vi "Get_MachineCode.vi"(8 "error in (no error)":errorcluster, 11 "Ref In":T1={"MS SQL Connection"=refnum, "UDL File"=path "", "Time"="", "DCODE"="", "WIP+1"=0, "MC No?"=0, "POKAYOKE?"=FALSE, "Expected Result"="", "Result [Status]"="", "Clock"=0.0, "RFID"="", "WIP Queue"=refnum, "TS Parameter"={"ProfitCenterCode"="", "LineCode"="", "WorkOrderNumber"="", "Model"="", "Model_with_Prefix"="", "VendorCode"="", "SetParameterDateCode"="", "PokaYoke"=0, "Target"=1, "Live_DateCode"="", "CustomerPartNumber"="", "Hand"="", "sBarcode"=FALSE, "FCA"=0, "Ent_Stamp"=timestamp(0 s since 1904-01-01), "STS_CD"=0.0}, "Data_Queue"=[], "RFID Serial No."=""} {"TS Parameter"."FCA" format="%01d"; "TS Parameter"."Target" min=1 max=100000; "TS Parameter"."PokaYoke" min=0 max=1}) -> (0 "error out":errorcluster, 1 "OperationCode":string[](array[string]), 2 "Machine Codes":string[](array[string]), 3 "Ref Out":T1={"MS SQL Connection"=refnum, "UDL File"=path "", "Time"="", "DCODE"="", "WIP+1"=0, "MC No?"=0, "POKAYOKE?"=FALSE, "Expected Result"="", "Result [Status]"="", "Clock"=0.0, "RFID"="", "WIP Queue"=refnum, "TS Parameter"={"ProfitCenterCode"="", "LineCode"="", "WorkOrderNumber"="", "Model"="", "Model_with_Prefix"="", "VendorCode"="", "SetParameterDateCode"="", "PokaYoke"=0, "Target"=1, "Live_DateCode"="", "CustomerPartNumber"="", "Hand"="", "sBarcode"=FALSE, "FCA"=0, "Ent_Stamp"=timestamp(0 s since 1904-01-01), "STS_CD"=0.0}, "Data_Queue"=[], "RFID Serial No."=""} {"TS Parameter"."FCA" format="%01d"; "TS Parameter"."Target" min=1 max=100000; "TS Parameter"."PokaYoke" min=0 max=1})   [LabVIEW 2020]
uses:
  Controls/TD SQL.ctl
  <vilib>/addons/database/Connection.llb/Conn ObjectReference.ctl
  Controls/WIP_State.ctl
  Controls/TS_Parameter.ctl
  <vilib>/regexp/Match Regular Expression.xnode
  <vilib>/addons/database/NI_Database_API.lvlib
panel:
  out "tables":string[](array[string])
  out "Array 2":string[](array[string])
  out "tables 2":string[](array[string])
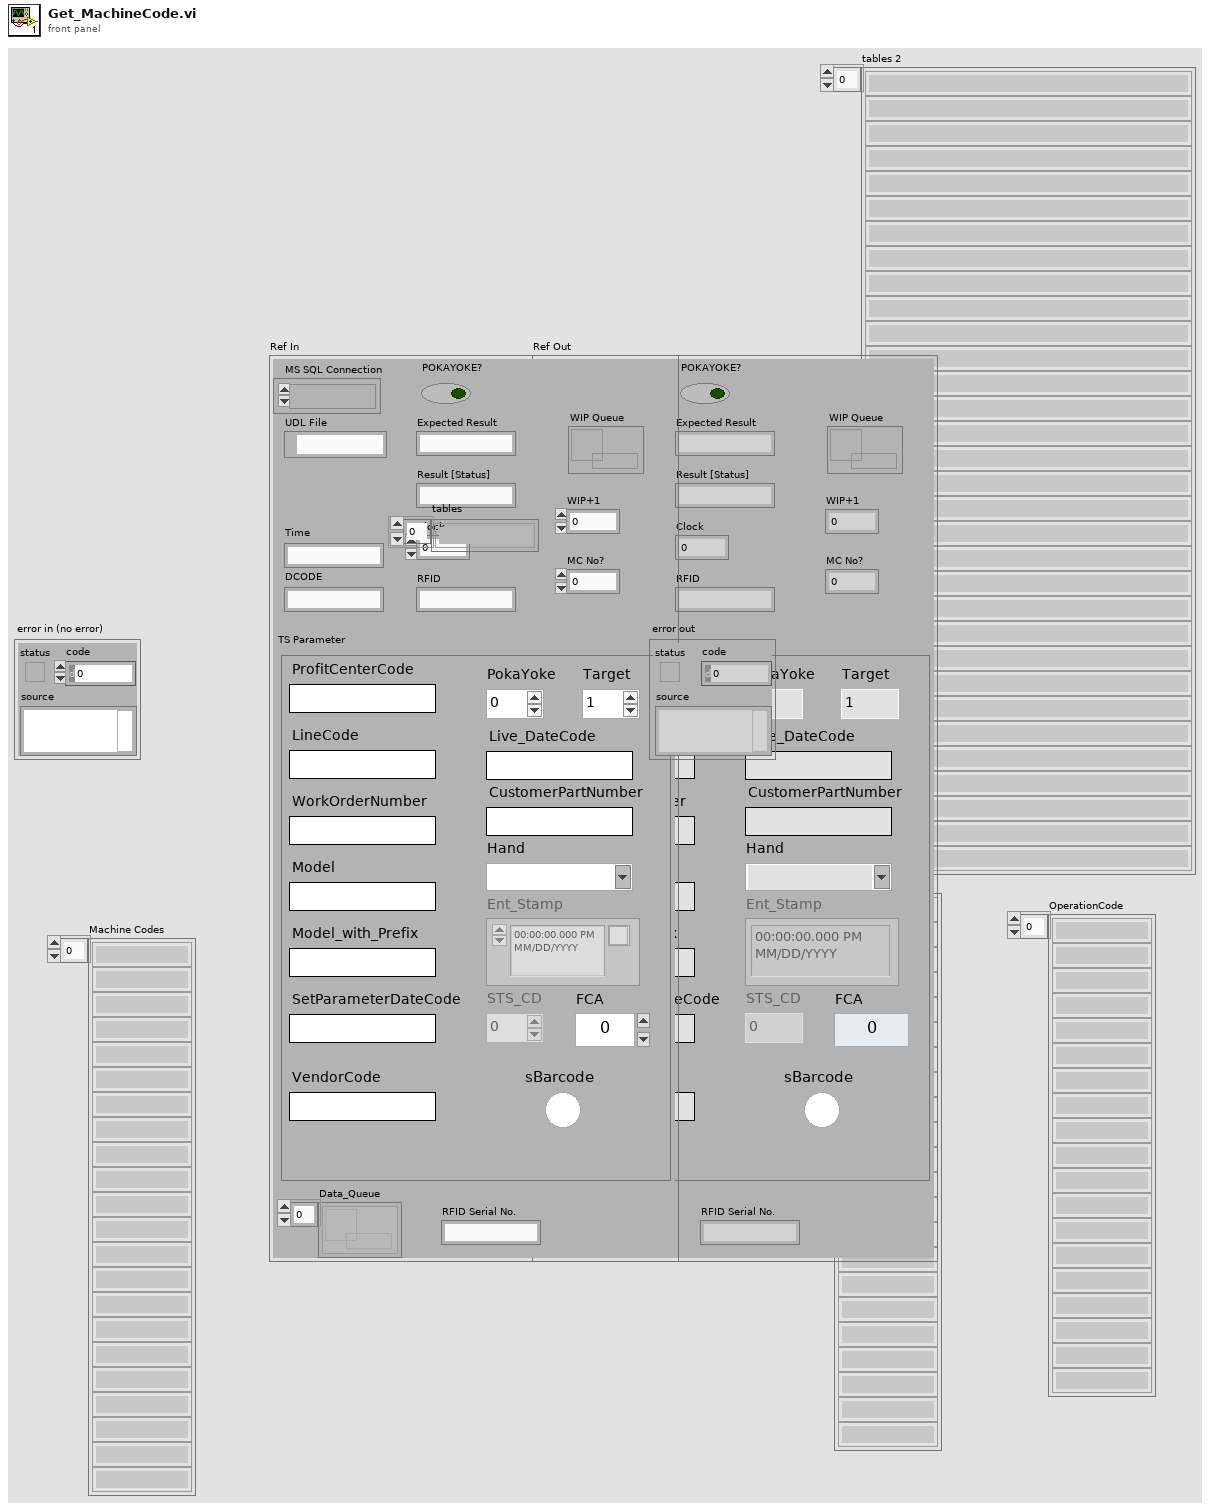
[diagram p1: front panel]
types:
  T1 = typedef "TD SQL.ctl" = cluster{"MS SQL Connection":T2, "UDL File":path, "Time":string, "DCODE":string, "WIP+1":i64, "MC No?":i32, "POKAYOKE?":bool, "Expected Result":string, "Result [Status]":string, "Clock":dbl, "RFID":string, "WIP Queue":refnum<queue>, "TS Parameter":T3, "Data_Queue":refnum<queue>[], "RFID Serial No.":string}
  T2 = typedef "NI_Database_API.lvlib/Conn ObjectReference.ctl" = refnum<k1>
  T3 = typedef "TS_Parameter.ctl" = cluster{"ProfitCenterCode":string, "LineCode":string, "WorkOrderNumber":string, "Model":string, "Model_with_Prefix":string, "VendorCode":string, "SetParameterDateCode":string, "PokaYoke":i32, "Target":i32, "Live_DateCode":string, "CustomerPartNumber":string, "Hand":string, "sBarcode":bool, "FCA":i32, "Ent_Stamp":timestamp, "STS_CD":dbl}
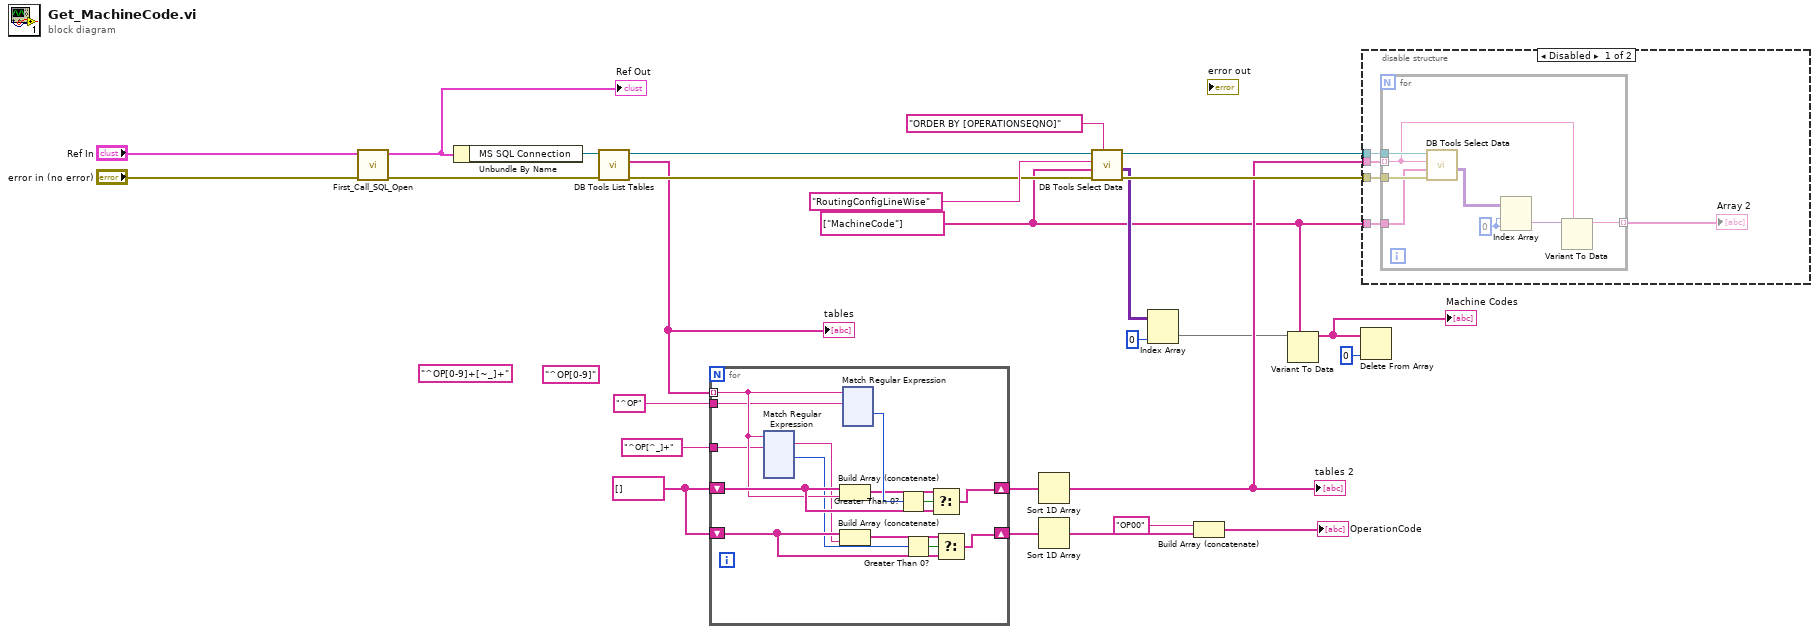
[diagram p0: block diagram]
diagram:
  (unwired) "^OP[0-9]" ("regular expression")
  (unwired) "^OP[0-9]+[~_]+" ("regular expression")
  w14 = string[] ["MachineCode"] ("columns")
  w6 = string[] [] ("tables")
  n1 = call "First_Call_SQL_Open.vi"("error in (no error)"="error in (no error)", "Ref In"="Ref In") -> ("error out"=w24:errorcluster, "Ref Out"=w26:T1)  [unwired: 8 in]
  "Ref Out" <- w26
  n2 = Unbundle By Name(w26) -> ("MS SQL Connection"=w25:T2)
  n3 = call <vilib>:"DB Tools List Tables.vi"("error in (no error)"=w24, "connection reference"=w25) -> ("error out"=w21:errorcluster, "tables"=w12:string[], "connection reference out"=w23:T2)  [unwired: 3 in]
  "tables" <- w12
  n4 = for {
    tunnel: w12 -> [w36] mode=indexing
    shift-right: [w37] -> w27
    shift-left: w6 -> [w38]
    tunnel: "^OP[^_]+" ("regular expression") -> [w35]
    shift-right: [w34] -> w5
    shift-left: w6 -> [w31]
    tunnel: "^OP" ("regular expression") -> [w28]
    n5 = xnode "Match Regular Expression"("input string"=w36, "regular expression"=w35) -> ("whole match"=w29:string, "offset past match"=w30:i32)  [unwired: 4 in, 4 out]
    n6 = Build Array (concatenate)(w38, w36) -> (w39:string[])
    n7 = Build Array (concatenate)(w31, w29) -> (w33:string[])
    n8 = xnode "Match Regular Expression"("input string"=w36, "regular expression"=w28) -> ("offset past match"=w41:i32)  [unwired: 4 in, 4 out]
    n9 = Greater Than 0?(x=w41) -> (x > 0?=w40:bool)
    n10 = Greater Than 0?(x=w30) -> (x > 0?=w32:bool)
    n11 = Select(t=w39, s=w40, f=w38) -> (s? t:f=w37:string[])
    n12 = Select(t=w33, s=w32, f=w31) -> (s? t:f=w34:string[])
  }
  n13 = Sort 1D Array(array=w27) -> (sorted array=w18:string[])
  "tables 2" <- w18
  n14 = Sort 1D Array(array=w5) -> (sorted array=w4:string[])
  n15 = call <vilib>:"DB Tools Select Data.vi"("condition"="ORDER BY [OPERATIONSEQNO]", "error in (no error)"=w21, "columns"=w14, "table"="RoutingConfigLineWise", "connection reference"=w23) -> ("error out"=w19:errorcluster, "data"=w16:variant[][], "connection reference out"=w20:T2)  [unwired: 1 in]
  n16 = Index Array(array=w16, index (col)=0 ("disabled index (col)")) -> (element=w15:variant[])  [unwired: 1 in]
  n17 = Build Array (concatenate)("OP00" ("String"), w4) -> (→"OperationCode":string[])
  n18 = Variant To Data(type=w14, Variant=w15) -> (data=w8:string[])  [unwired: 1 in, 1 out]
  "Machine Codes" <- w8
  n19 = Delete From Array(array=w8, index=0) -> ()  [unwired: 1 in, 2 out]
  n20 = disable-structure shown="Disabled" {
    disable-tunnel: w20 -> [w276 _]
    disable-tunnel: w19 -> [w275 _]
    disable-tunnel: w18 -> [w274 _]
    disable-tunnel: w14 -> [w273 _]
    frame Disabled {
      n21 = for {
        tunnel: w276 -> [w284]
        tunnel: w275 -> [w283]
        tunnel: w274 -> [w277] mode=indexing
        tunnel: w273 -> [w280]
        tunnel: [w279] -> w272 mode=indexing
        w278 = 0 ("disabled index (col)")
        n22 = call <vilib>:"DB Tools Select Data.vi"("error in (no error)"=w283, "columns"=w280, "table"=w277, "connection reference"=w284) -> ("data"=w282:variant[][])  [unwired: 2 in, 2 out]
        n23 = Index Array(array=w282, index (row)=w278, index (col)=w278) -> (element=w281:variant)
        n24 = Variant To Data(type=w277, Variant=w281) -> (data=w279:string)  [unwired: 1 in, 1 out]
      }
      "Array 2" <- w272
    }
    frame Enabled {
    }
  }
